vi "Launcher.vi"() -> ()   [LabVIEW 2020]
doc: "Launcher para seleccionar entre cual marca de micro usar y su puerto com"
uses:
  Abstract/Serial Device/Control 1.ctl
  UI Actor/UI Actor.lvclass
  C:/Program Files (x86)/National Instruments/LabVIEW 2020/vi.lib/ActorFramework/Actor/Actor.lvclass
  UI Actor/UI Actor.lvclass/UI Actor.ctl
  UI Actor/Write Visa com port 2.vi
  UI Actor/Write Marca.vi
  <vilib>/ActorFramework/Actor/Actor.lvclass
panel:
  in  "Marca":T1
  in  "Visa com port":refnum<visa-resource-name>
  # "BIENVENIDO"
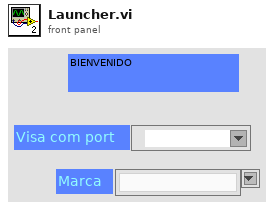
[diagram p1: front panel]
types:
  T1 = typedef "Control 1.ctl" = string
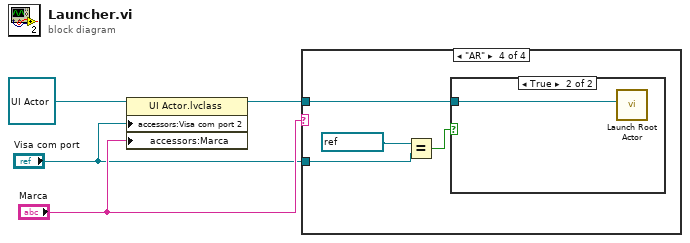
[diagram p0: block diagram]
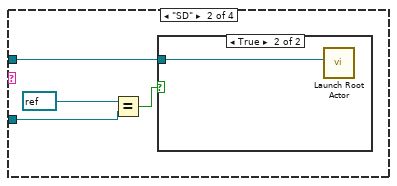
[diagram p3: hidden frame]
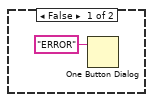
[diagram p4: hidden frame]
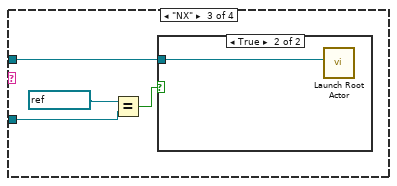
[diagram p5: hidden frame]
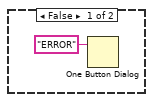
[diagram p6: hidden frame]
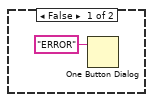
[diagram p7: hidden frame]
diagram:
  n1 = property class="UI Actor.lvclass"(reference=refnum<class "UI Actor.lvclass"> refnum ("UI Actor.lvlib:UI Actor.lvclass"), "accessors:Visa com port 2"="Visa com port", "accessors:Marca"="Marca") -> (reference out=w3:refnum<class "UI Actor.lvclass">)  [unwired: 1 in, 1 out]
  n2 = case shown="\"AR\"" "Marca" {
    tunnel: w3 -> [_ w8 w14 w20]
    tunnel: "Visa com port" -> [_ w7 w13 w19]
    frame "False", Default {
    }
    frame "SD" {
      n3 = Equal?(x=refnum<visa-resource-name> refnum, y=w7) -> (x = y?=w5:bool)
      n4 = case shown="True" w5 {
        tunnel: w8 -> [_ w10]
        frame False {
          n5 = One Button Dialog(message="ERROR") -> ()  [unwired: 1 in, 1 out]
        }
        frame True {
          n6 = call <vilib>:"Launch Root Actor.vi"("Actor"=w10) -> ()  [unwired: 9 in, 2 out]
        }
      }
    }
    frame "NX" {
      n7 = Equal?(x=refnum<visa-resource-name> "COM3", y=w13) -> (x = y?=w11:bool)
      n8 = case shown="True" w11 {
        tunnel: w14 -> [_ w16]
        frame False {
          n9 = One Button Dialog(message="ERROR") -> ()  [unwired: 1 in, 1 out]
        }
        frame True {
          n10 = call <vilib>:"Launch Root Actor.vi"("Actor"=w16) -> ()  [unwired: 9 in, 2 out]
        }
      }
    }
    frame "AR" {
      n11 = Equal?(x=refnum<visa-resource-name> "COM5", y=w19) -> (x = y?=w17:bool)
      n12 = case shown="True" w17 {
        tunnel: w20 -> [_ w22]
        frame False {
          n13 = One Button Dialog(message="ERROR") -> ()  [unwired: 1 in, 1 out]
        }
        frame True {
          n14 = call <vilib>:"Launch Root Actor.vi"("Actor"=w22) -> ()  [unwired: 9 in, 2 out]
        }
      }
    }
  }
